vi "DeviceOn.vi"(8 "error in (no error)":errorcluster, 11 "NHRDCPower in":refnum<class "NHRDCPower.lvclass">) -> (0 "error out":errorcluster, 3 "NHRDCPower out":refnum<class "NHRDCPower.lvclass">)   [LabVIEW 2018, in "AcPwrPlugins.lvlib" / "NHRDCPower.lvclass"]
doc: "This VI enables the instruments output to either generate or recieving a signal."
uses:
  NHRDCPower.lvclass
  <vilib>/ErrorRing/Error Ring.xnode
  <instrlib>/NHRDCPowerModule/NHRDCPowerModule/NHRDCPowerModule.lvlib
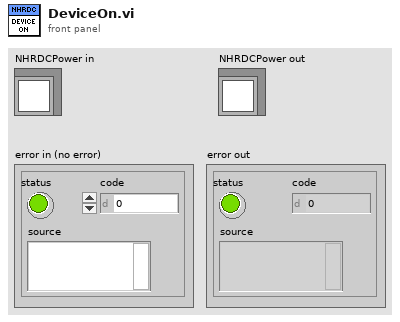
[diagram p1: front panel]
types:
  T1 = typedef "AcPwrPlugins.lvlib/NHRDCPower.lvclass/Device(s)Settings.ctl" = cluster{"Handle":string, "Name":string, "id query (Yes)":bool, "reset device (Yes)":bool, "Connected":bool, "Voltage Range (V)":dbl[], "Timing":cluster{"TimingOn":enum16{""}, "Hours":u32, "Minutes":u32, "Seconds":dbl, "CutoffVoltage":dbl}, "Initial Battery Detect Voltage (0)":sgl, "SafetySettings":cluster{"SetWatchDog":bool, "Voltage (V)":sgl, "Current (A)":sgl, "Power (W)":sgl, "Voltage Delay (s)":sgl, "Current Delay (s)":sgl, "Power Delay (s)":sgl}, "Options String":string, "Aperture Time (s)":sgl, "operating state (Off)":i32, "OutputSettings":cluster{"Voltage (V)":sgl, "Current (A)":sgl, "Resistance (Ohms)":sgl, "Power (W)":sgl, "Enable Voltage":bool, "Enable Current":bool, "Enable Resistance":bool, "Enable Power":bool, "Delay After (s)":sgl}[], "SlewRate":cluster{"Set Voltage Rate V/S":sgl, "Set Current Rate A/S":sgl, "Set Resistance Rate R/S":sgl, "Set Power Rate W/S":sgl}}[]
  T2 = cluster{"Voltage (V)":sgl, "Current (A)":sgl, "Resistance (Ohms)":sgl, "Power (W)":sgl, "Enable Voltage":bool, "Enable Current":bool, "Enable Resistance":bool, "Enable Power":bool, "Delay After (s)":sgl}[]
  T3 = cluster{"Voltage (V)":sgl, "Current (A)":sgl, "Resistance (Ohms)":sgl, "Power (W)":sgl, "Enable Voltage":bool, "Enable Current":bool, "Enable Resistance":bool, "Enable Power":bool, "Delay After (s)":sgl}
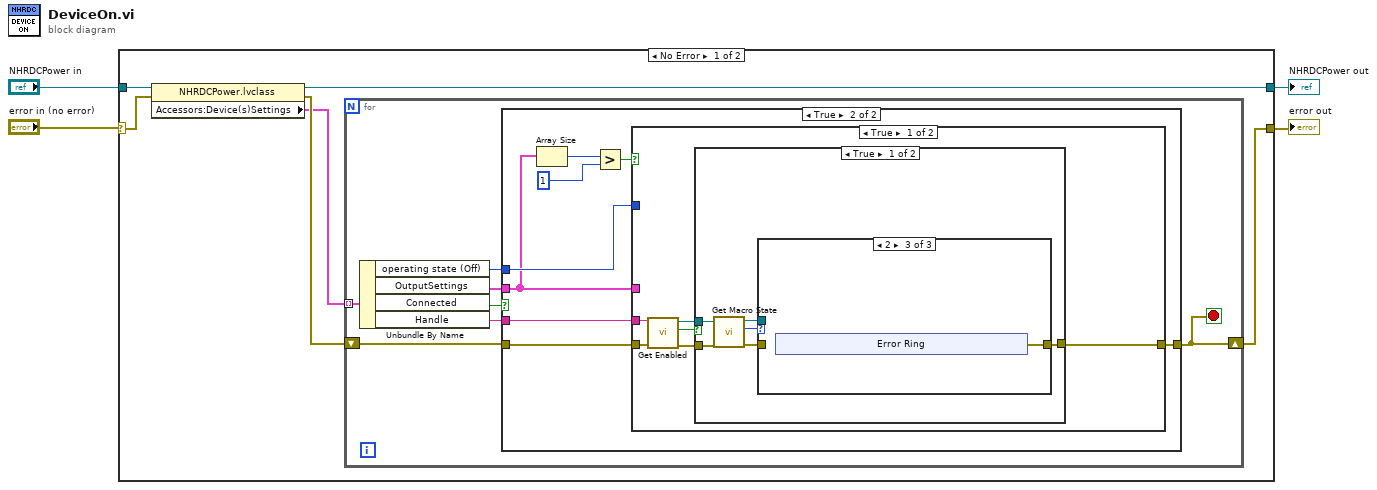
[diagram p0: block diagram]
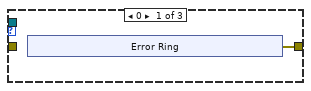
[diagram p3: hidden frame]
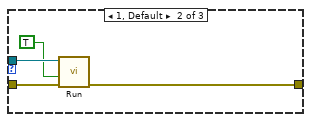
[diagram p4: hidden frame]
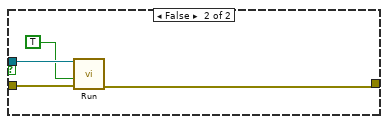
[diagram p5: hidden frame]
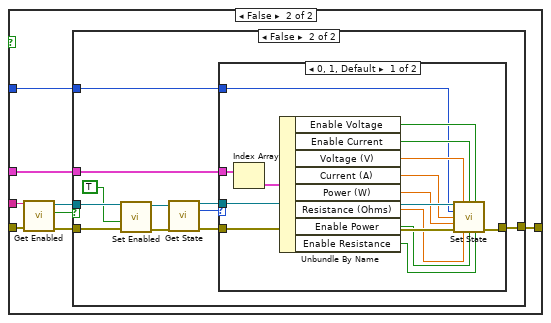
[diagram p6: hidden frame]
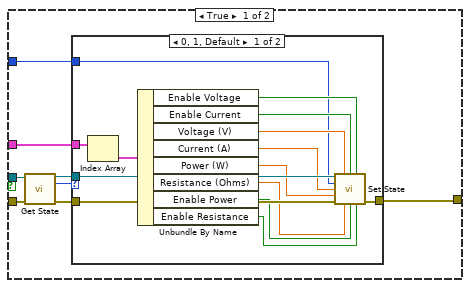
[diagram p7: hidden frame]
diagram:
  n1 = case shown="No Error" "error in (no error)" {
    selector: "error in (no error)" -> [w9 w109]
    tunnel: [w8 w109] -> w1
    tunnel: [w10 w108] -> w3
    tunnel: "NHRDCPower in" -> [w6 w108]
    frame No Error {
      n2 = property class="NHRDCPower.lvclass"(reference=w6, error in=w9) -> (reference out=w10:refnum<class "NHRDCPower.lvclass">, error out=w7:errorcluster, "Accessors:Device(s)Settings"=w5:T1)
      n3 = for {
        tunnel: w5 -> [w17] mode=indexing
        shift-right: [w15] -> w8
        shift-left: w7 -> [w16]
        stop <- w15 stop-if-true
        n4 = Unbundle By Name(w17) -> ("operating state (Off)"=w11:i32, "OutputSettings"=w12:T2, "Connected"=w13:bool, "Handle"=w14:string)
        n5 = case shown="True" w13 {
          tunnel: w16 -> [w18 w25]
          tunnel: [w18 w26] -> w15
          tunnel: w14 -> [_ w24]
          tunnel: w12 -> [_ w22]
          tunnel: w11 -> [_ w23]
          frame False {
          }
          frame True {
            n6 = Array Size(array=w22) -> (size(s)=w21:i32)
            n7 = Greater?(x=w21, y=1) -> (0:w19:bool)
            n8 = case shown="True" w19 {
              tunnel: [w32 w58] -> w26
              tunnel: w25 -> [w31 w57]
              tunnel: w24 -> [w30 w56]
              tunnel: w23 -> [_ w52]
              tunnel: w22 -> [_ w51]
              frame True {
                n9 = call <instrlib>:"Get Enabled.vi"("error in (no error)"=w31, "instrument handle"=w30) -> ("error out"=w29:errorcluster, "enabled"=w27:bool, "instrument handle out"=w28:refnum<visa-resource-name>)  [unwired: 7 in]
                n10 = case shown="True" w27 {
                  tunnel: [w35 w48] -> w32
                  tunnel: w29 -> [w38 w49]
                  tunnel: w28 -> [w37 w50]
                  frame True {
                    n11 = call <instrlib>:"Get Macro State.vi"("error in (no error)"=w38, "instrument handle"=w37) -> ("error out"=w36:errorcluster, "state"=w33:i32, "instrument handle out"=w34:refnum<visa-resource-name>)  [unwired: 7 in]
                    n12 = case shown="2" w33 {
                      tunnel: w36 -> [_ w44 _]
                      tunnel: [w39 w41 w45] -> w35
                      tunnel: w34 -> [_ w43 _]
                      frame 0 {
                        n13 = xnode "Error Ring"() -> ("error out"=w39:errorcluster)
                      }
                      frame 1, Default {
                        n14 = call <instrlib>:"Run.vi"("error in (no error)"=w44, "continuous (false)"=TRUE, "instrument handle"=w43) -> ("error out"=w41:errorcluster)  [unwired: 7 in, 1 out]
                      }
                      frame 2 {
                        n15 = xnode "Error Ring"() -> ("error out"=w45:errorcluster)
                      }
                    }
                  }
                  frame False {
                    n16 = call <instrlib>:"Run.vi"("error in (no error)"=w49, "continuous (false)"=TRUE, "instrument handle"=w50) -> ("error out"=w48:errorcluster)  [unwired: 7 in, 1 out]
                  }
                }
              }
              frame False {
                n17 = call <instrlib>:"Get Enabled.vi"("error in (no error)"=w57, "instrument handle"=w56) -> ("error out"=w55:errorcluster, "enabled"=w53:bool, "instrument handle out"=w54:refnum<visa-resource-name>)  [unwired: 7 in]
                n18 = case shown="False" w53 {
                  tunnel: [w66 w92] -> w58
                  tunnel: w55 -> [w65 w85]
                  tunnel: w54 -> [w64 w86]
                  tunnel: w51 -> [w60 w83]
                  tunnel: w52 -> [w59 w82]
                  frame True {
                    n19 = call <instrlib>:"Get State.vi"("instrument handle"=w64, "error in (no error)"=w65) -> ("instrument handle out"=w61:refnum<visa-resource-name>, "operating state"=w62:i32, "error out"=w63:errorcluster)  [unwired: 3 in, 8 out]
                    n20 = case shown="0, 1, Default" w62 {
                      tunnel: [w79 w81] -> w66
                      tunnel: w63 -> [w80 w81]
                      tunnel: w61 -> [w77 _]
                      tunnel: w60 -> [w78 _]
                      tunnel: w59 -> [w67 _]
                      frame 0, 1, Default {
                        n21 = Index Array(array=w78) -> (element=w68:T3)  [unwired: 1 in]
                        n22 = Unbundle By Name(w68) -> ("Enable Voltage"=w69:bool, "Enable Current"=w70:bool, "Voltage (V)"=w71:sgl, "Current (A)"=w72:sgl, "Power (W)"=w73:sgl, "Resistance (Ohms)"=w74:sgl, "Enable Power"=w75:bool, "Enable Resistance"=w76:bool)
                        n23 = call <instrlib>:"Set State.vi"("instrument handle"=w77, "voltage (0.0)"=w71, "current enabled (false)"=w70, "voltage enabled (false)"=w69, "operating state (Off)"=w67, "current (0.0)"=w72, "power (0.0)"=w73, "error in (no error)"=w80, "resistance (0.0)"=w74, "power enabled (false)"=w75, "resistance enabled (false)"=w76) -> ("error out"=w79:errorcluster)  [unwired: 3 in, 1 out]
                      }
                      frame 2..4 {
                      }
                    }
                  }
                  frame False {
                    n24 = call <instrlib>:"Set Enabled.vi"("error in (no error)"=w85, "enabled (false)"=TRUE, "instrument handle"=w86) -> ("error out"=w88:errorcluster, "instrument handle out"=w87:refnum<visa-resource-name>)  [unwired: 7 in]
                    n25 = call <instrlib>:"Get State.vi"("instrument handle"=w87, "error in (no error)"=w88) -> ("instrument handle out"=w89:refnum<visa-resource-name>, "operating state"=w90:i32, "error out"=w91:errorcluster)  [unwired: 3 in, 8 out]
                    n26 = case shown="0, 1, Default" w90 {
                      tunnel: [w105 w107] -> w92
                      tunnel: w91 -> [w106 w107]
                      tunnel: w89 -> [w104 _]
                      tunnel: w83 -> [w95 _]
                      tunnel: w82 -> [w93 _]
                      frame 0, 1, Default {
                        n27 = Index Array(array=w95) -> (element=w94:T3)  [unwired: 1 in]
                        n28 = Unbundle By Name(w94) -> ("Enable Voltage"=w96:bool, "Enable Current"=w97:bool, "Voltage (V)"=w98:sgl, "Current (A)"=w99:sgl, "Power (W)"=w100:sgl, "Resistance (Ohms)"=w101:sgl, "Enable Power"=w102:bool, "Enable Resistance"=w103:bool)
                        n29 = call <instrlib>:"Set State.vi"("instrument handle"=w104, "voltage (0.0)"=w98, "current enabled (false)"=w97, "voltage enabled (false)"=w96, "operating state (Off)"=w93, "current (0.0)"=w99, "power (0.0)"=w100, "error in (no error)"=w106, "resistance (0.0)"=w101, "power enabled (false)"=w102, "resistance enabled (false)"=w103) -> ("error out"=w105:errorcluster)  [unwired: 3 in, 1 out]
                      }
                      frame 2..4 {
                      }
                    }
                  }
                }
              }
            }
          }
        }
      }
    }
    frame Error {
    }
  }
  "error out" <- w1
  "NHRDCPower out" <- w3
